vi "Write plugins.vi"(8 "error in (no error)":errorcluster, 10 "plugins":cluster{"id":string, "values":T1}[](array[cluster]), 11 "DSFConfiguration in":refnum<class "DSFConfiguration.lvclass">) -> (0 "error out":errorcluster, 3 "DSFConfiguration out":refnum<class "DSFConfiguration.lvclass">)   [LabVIEW 2017, in "DSFConfiguration.lvclass"]
uses:
  DSFConfiguration.lvclass
  Controls/dsf configuration file/1.0.0/dsf timing.ctl
  Controls/dsf configuration file/1.0.0/dsf plugin.ctl
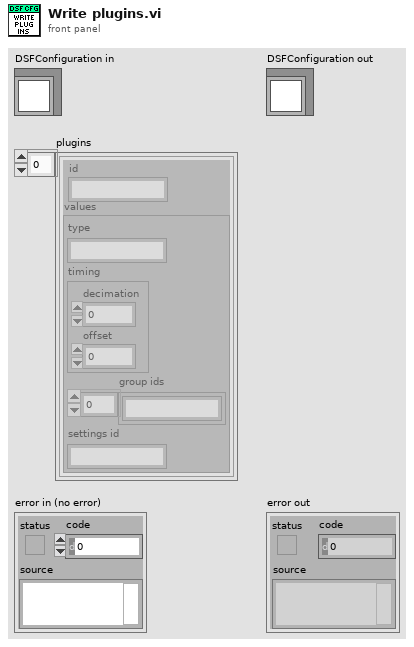
[diagram p1: front panel]
types:
  T1 = typedef "dsf configuration file v1.0.0.lvlib/dsf plugin.ctl" = cluster{"type":string, "timing":T2, "group ids":string[], "settings id":string}
  T2 = typedef "dsf configuration file v1.0.0.lvlib/dsf timing.ctl" = cluster{"decimation":i32, "offset":i32}
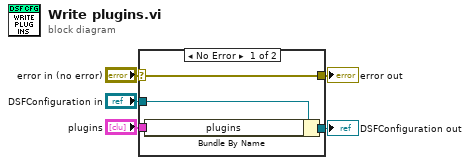
[diagram p0: block diagram]
diagram:
  n1 = case shown="No Error" "error in (no error)" {
    selector: "error in (no error)" -> [w9 w10]
    tunnel: [w9 w10] -> w4
    tunnel: [w7 w11] -> w2
    tunnel: "DSFConfiguration in" -> [w8 w11]
    tunnel: "plugins" -> [w6 _]
    frame No Error {
      n2 = Bundle By Name(cluster=w8, "plugins"=w6) -> (w7:refnum<class "DSFConfiguration.lvclass">)
    }
    frame Error {
    }
  }
  "error out" <- w4
  "DSFConfiguration out" <- w2
